vi "execute.vi"(8 "error in (no error)":errorcluster, 9 "image assembler in":refnum<class "GenericComponent.lvclass">, 10 "imaging mode in":refnum<class "GenericComponent.lvclass">, 11 "AdapterCN091113ImagingModeToImageAssembler in":refnum<class "AdapterCN091113ImagingModeToImageAssembler.lvclass">) -> (0 "error out":errorcluster, 1 "image assembler out":refnum<class "GenericComponent.lvclass">, 2 "imaging mode out":refnum<class "GenericComponent.lvclass">, 3 "AdapterCN091113ImagingModeToImageAssembler out":refnum<class "AdapterCN091113ImagingModeToImageAssembler.lvclass">)   [LabVIEW 2010, in "AdapterCN091113ImagingModeToImageAssembler.lvclass"]
uses:
  AdapterCN091113ImagingModeToImageAssembler.lvclass
  common/classes/GenericComponent/GenericComponent/GenericComponent.lvclass
  ImagingMode/ImagingModeDL100901FlexTrajectory/ImagingModeDL100901FlexTrajectory/ImagingModeDL100901FlexTrajectory.lvclass
  ImageAssembler/ImageAssemblerDL090211Frame/ImageAssemblerDL090211Frame/ImageAssemblerDL090211Frame.lvclass
  Trajectory/GenericTrajectory/GenericTrajectory/GenericTrajectory.lvclass
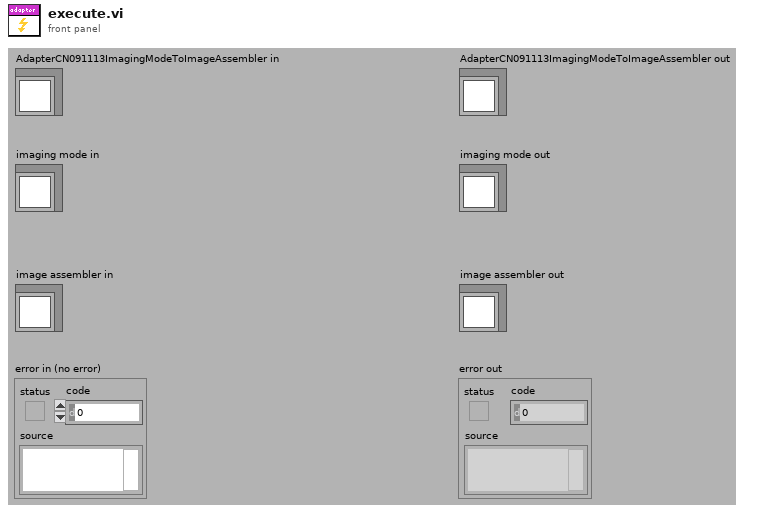
[diagram p1: front panel]
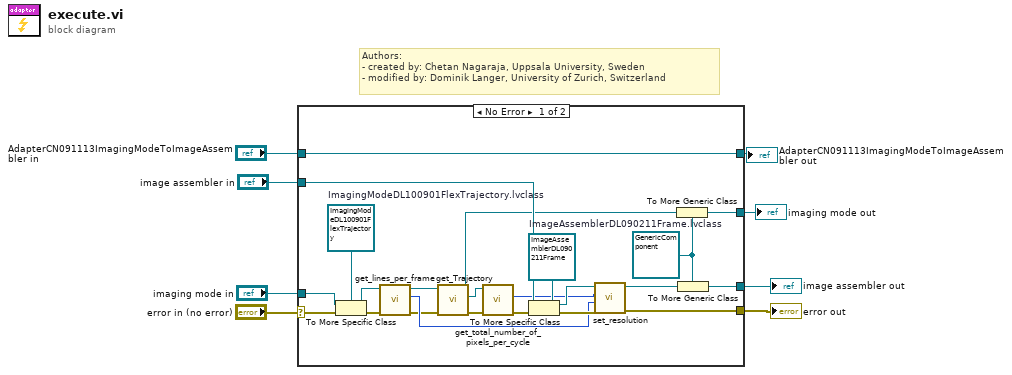
[diagram p0: block diagram]
diagram:
  # "Authors: \n- created by: Chetan Nagaraja, Uppsala University, Sweden\n- modified by: Dominik Langer, University of Zurich, Switzerland"
  n1 = case shown="No Error" "error in (no error)" {
    selector: "error in (no error)" -> [w31 w34]
    tunnel: "imaging mode in" -> [w30 w32]
    tunnel: "image assembler in" -> [w28 w33]
    tunnel: [w24 w34] -> w5
    tunnel: [w22 w33] -> w4
    tunnel: [w21 w32] -> w3
    tunnel: "AdapterCN091113ImagingModeToImageAssembler in" -> [w20 w35]
    tunnel: [w20 w35] -> w1
    frame No Error {
      w19 = refnum<class "ImagingModeDL100901FlexTrajectory.lvclass"> refnum  # ImagingModeDL100901FlexTrajectory.lvclass
      w25 = refnum<class "GenericComponent.lvclass"> refnum ("GenericComponent.lvclass")
      w29 = refnum<class "ImageAssemblerDL090211Frame.lvclass"> refnum  # ImageAssemblerDL090211Frame.lvclass
      n2 = To More Specific Class(target class=w19, reference=w30, error in=w31) -> (specific class reference=w17:refnum<class "ImagingModeDL100901FlexTrajectory.lvclass">, error out=w18:errorcluster)
      n3 = call-dynamic "get_lines_per_frame.vi"("error in (no error)"=w18, "ScanModeCN090721ThreeDScan in"=w17) -> ("error out"=w15:errorcluster, "lines per frame"=w16:i32, "ScanModeCN090721ThreeDScan out"=w12:refnum<class "ImagingModeDL100901FlexTrajectory.lvclass">)  [unwired: 7 in]
      n4 = call-dynamic "get_Trajectory.vi"("error in (no error)"=w15, "ScanModeDL090923Scaffold in"=w12) -> ("error out"=w13:errorcluster, "Trajectory"=w10:refnum<class "GenericTrajectory.lvclass">, "ScanModeDL090923Scaffold out"=w11:refnum<class "ImagingModeDL100901FlexTrajectory.lvclass">)  [unwired: 2 in, 5 out]
      n5 = call-dynamic "get_total_number_of_pixels_per_cycle.vi"("error in (no error)"=w13, "GenericTrajectory in"=w10) -> ("error out"=w14:errorcluster, "total number of pixels per cycle"=w9:i32)  [unwired: 7 in, 1 out]
      n6 = To More Specific Class(target class=w29, reference=w28, error in=w14) -> (specific class reference=w26:refnum<class "ImageAssemblerDL090211Frame.lvclass">, error out=w27:errorcluster)
      n7 = call "set_resolution.vi"("error in (no error)"=w27, "y resolution"=w16, "x resolution"=w9, "DL090211FrameImageAssembler.lvclass in"=w26) -> ("error out"=w24:errorcluster, "DL090211FrameImageAssembler.lvclass out"=w23:refnum<class "ImageAssemblerDL090211Frame.lvclass">)  [unwired: 6 in]
      n8 = To More Generic Class(target class=w25, reference=w11) -> (generic class reference=w21:refnum<class "GenericComponent.lvclass">)
      n9 = To More Generic Class(target class=w25, reference=w23) -> (generic class reference=w22:refnum<class "GenericComponent.lvclass">)
    }
    frame Error {
    }
  }
  "error out" <- w5
  "AdapterCN091113ImagingModeToImageAssembler out" <- w1
  "imaging mode out" <- w3
  "image assembler out" <- w4
